vi "Discovery Engine.vi"() -> ()   [LabVIEW 2020]
doc: "This VI broadcasts the IP addresses available on the target on the UDP broadcast address 234.5.6.7, port 58432. It sends this data wrapped in the generic data frame."
uses:
  Type Definitions/Data Frame.ctl
  Type Definitions/Data Frame Header.ctl
  Type Definitions/Payload Class.ctl
  Type Definitions/Device.ctl
  Type Definitions/Discovery Engine State.ctl
  <vilib>/Platform/TimedLoop/XDataNode/timing_clust.ctl
  <vilib>/Platform/TimedLoop/XDataNode/nitl_modes.ctl
  <vilib>/Platform/TimedLoop/XDataNode/wakeup.ctl
  Type Definitions/Network Adapter State.ctl
  Type Definitions/Enum - System State.ctl
  <vilib>/Utility/tcp.llb/UDP Multicast Write-Only Open.vi
  <vilib>/platform/TimedLoop/XDataNode/XDataNode.xnode
  <vilib>/Platform/TimedLoop/XDataNode/XDNodeRunTimeDep.lvlib
panel:
  out "Notifier":refnum<notifier>
  out "Frame":T1 {"CRC" format="%08x"; "Frame Header"."Options" format="%016b"; "Frame Header"."Time" format="%^<%I:%M:%S%3u %p\n%m/%d/%Y %Z>T"; "Frame Header"."Sync" format="%08x"}
  out "Valid IP Addresses":i32
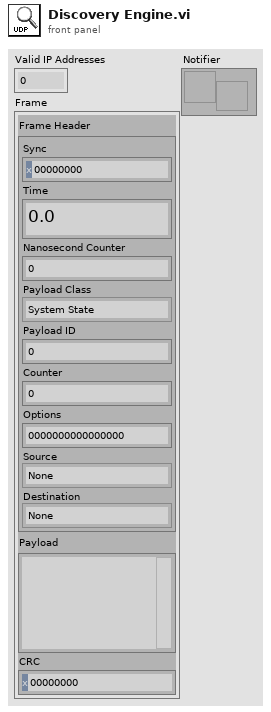
[diagram p1: front panel]
types:
  T1 = typedef "Data Frame.ctl" = cluster{"Frame Header":T2, "Payload":string, "CRC":u32}
  T2 = typedef "Data Frame Header.ctl" = cluster{"Sync":u32, "Time":dbl, "Nanosecond Counter":i64, "Payload Class":T3, "Payload ID":u16, "Counter":i32, "Options":u32, "Source":T4, "Destination":T4}
  T3 = typedef "Payload Class.ctl" = enum16{"System State", "Parameters", "Metadata", "Software Monitor", "Data", "Commands"}
  T4 = typedef "Device.ctl" = enum32{"None", "Exec", "Aux1", "Aux2", "Aux3"}
  T5 = typedef "Discovery Engine State.ctl" = cluster{"Adapter IP Address":string, "Connection ID":refnum<k16>, "Error":errorcluster}
  T6 = typedef "XDNodeRunTimeDep.lvlib/timing_clust.ctl" = cluster{"Expected End [f-1]":u64, "Actual End [f-1]":u64, "Finished Late? [f-1]":bool, "Expected End [i-1]":u64, "Actual End [i-1]":u64, "Finished Late? [i-1]":bool, "Expected Start [i]":u64, "Actual Start [i]":u64, "Expected Start [f]":u64, "Actual Start [f]":u64, "Source Name":string, "Structure Name":string, "Period":i64, "Deadline":i64, "Offset":i64, "Start":i64, "Priority":i32, "Timeout":i32, "Mode":T7, "Wakeup Reason":T8, "Error":errorcluster, "Source Type":string, "Secondary Source Type":string, "Global End Time":u64, "Global Start Time":u64, "Frame Duration":u64, "Iteration Duration":u64, "Assigned CPU":i32, "I/O Scan Engine Mode":u32}
  T7 = typedef "XDNodeRunTimeDep.lvlib/nitl_modes.ctl" = enum32{"No Change", "Process missed periods, maintain original phase", "Discard missed periods, maintain original phase", "Process missed periods, ignore original phase", "Discard missed periods, ignore original phase"}
  T8 = typedef "XDNodeRunTimeDep.lvlib/wakeup.ctl" = enum32{"Normal", "Aborted", "Asynchronous wakeup", "Timing source error", "Timed loop error", "Timeout"}
  T9 = typedef "Enum - System State.ctl" = enum16{"System Time", "Telemetry TCP State", "Writeable Drive State", "Command TCP State", "Network Adapter State", "Discovery Engine State", "Disk State"}
  T10 = typedef "Network Adapter State.ctl" = cluster{"Adapter IP Addresses":string[]}
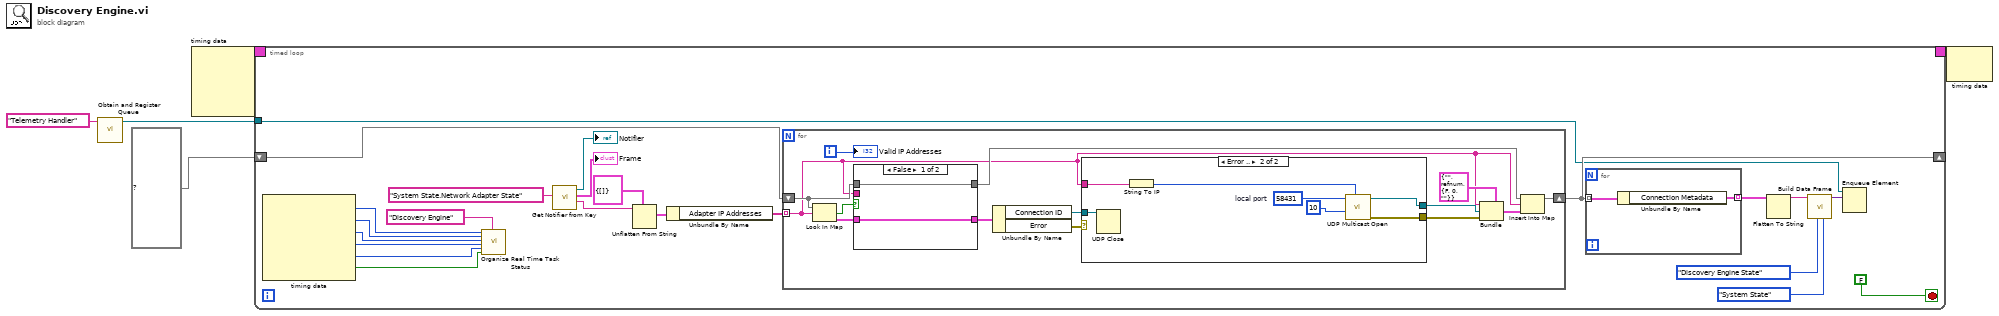
[diagram p0: block diagram]
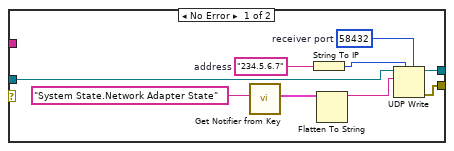
[diagram p2: hidden frame]
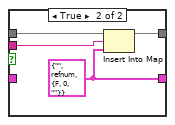
[diagram p3: hidden frame]
diagram:
  n1 = call "Obtain and Register Queue.vi"("name (unnamed)"="Telemetry Handler") -> ("Queue Out"=w3:refnum<queue>)  [unwired: 7 in, 3 out]
  n2 = node-c288() -> (w5:T6)  [unwired: 4 in]
  n3 = timed-loop {
    timing: w5 -> [_]
    timing-out: [_] -> w4
    tunnel: w3 -> [w9]
    shift-right: [w15] -> _
    shift-left: map{string, T5} {} ("map") -> [w16]
    stop <- FALSE stop-if-true
    n4 = node-c288() -> (w26:i32, w25:i32, w24:i64, w23:i64, w22:i64, w21:bool)  [unwired: 1 in]
    n5 = call "Organize Real Time Task Status.vi"("Priority"=w26, "Processor"=w25, "Offset"=w24, "Iteration Duration"=w23, "Period"=w22, "Finished Late? [i-1]"=w21, "Task Name"="Discovery Engine") -> ()  [unwired: 12 in, 1 out]
    n6 = call "Get Notifier from Key.vi"("Notifier Key"="System State.Network Adapter State") -> ("Payload"=w18:string, "Frame"=→"Frame":T1, "Notifier"=→"Notifier":refnum<notifier>)  [unwired: 8 in]
    n7 = Unflatten From String(type=T10 {"Adapter IP Addresses"=[]} ("Network Adapter Metadata"), binary string=w18) -> (value=w20:T10)  [unwired: 3 in, 2 out]
    n8 = Unbundle By Name(w20) -> ("Adapter IP Addresses"=w8:string[])
    n9 = for {
      tunnel: w8 -> [w31] mode=indexing
      shift-right: [w37] -> w15
      shift-left: w16 -> [w43]
      i -> [w34]
      n10 = Look In Map(map=w43, key=w31) -> (key not found?=w44:bool, value=w42:T5)  [unwired: 1 in]
      n11 = case shown="False" w44 {
        tunnel: w43 -> [w62 w66]
        tunnel: w31 -> [_ w65]
        tunnel: [w62 w64] -> w38
        tunnel: w42 -> [w61 _]
        tunnel: [w61 w63] -> w41
        frame False {
        }
        frame True {
          w63 = T5 {"Adapter IP Address"="", "Connection ID"=refnum, "Error"={"status"=FALSE, "code"=0, "source"=""}} ("Connection Metadata")
          n12 = Insert Into Map(map in=w66, key=w65, value=w63) -> (map out=w64:map{string, T5})  [unwired: 2 out]
        }
      }
      n13 = Unbundle By Name(w41) -> ("Connection ID"=w40:refnum<k16>, "Error"=w39:errorcluster)
      n14 = case shown="Error .." w39 {
        tunnel: [w51 w58] -> w33
        tunnel: [w50 w59] -> w32
        tunnel: w40 -> [w49 w60]
        tunnel: w31 -> [_ w54]
        frame No Error {
          w48 = u16 58432  # receiver port
          w46 = "234.5.6.7"  # address
          n15 = call "Get Notifier from Key.vi"("Notifier Key"="System State.Network Adapter State") -> ("Frame"=w52:T1)  [unwired: 8 in, 2 out]
          n16 = String To IP(1:w46) -> (0:w47:u32)
          n17 = Flatten To String(anything=w52) -> (data string=w45:string)  [unwired: 3 in, 2 out]
          n18 = UDP Write(address=w47, port or service name=w48, connection ID=w49, data in=w45) -> (error out=w51:errorcluster, 3:w50:refnum<k16>)  [unwired: 2 in]
        }
        frame Error {
          w57 = u16 58431  # local port
          n19 = UDP Close(connection ID=w60) -> ()  [unwired: 1 in, 2 out]
          n20 = String To IP(1:w54) -> (0:w55:u32)
          n21 = call-poly <vilib>:"UDP Multicast Open.vi"("net address"=w55, "time-to-live (1)"=u16 10, "port"=w57) -> ("error out"=w58:errorcluster, "connection ID"=w59:refnum<k16>)  [unwired: 7 in]
        }
      }
      n22 = Bundle(cluster=T5 {"Adapter IP Address"="", "Connection ID"=refnum, "Error"={"status"=FALSE, "code"=0, "source"=""}} ("Connection Metadata"), "Adapter IP Address"=w31, "Connection ID"=w32, "Error"=w33) -> (w36:T5)
      n23 = Insert Into Map(map in=w38, key=w31, value=w36) -> (map out=w37:map{string, T5})  [unwired: 2 out]
      "Valid IP Addresses" <- w34
    }
    n24 = for {
      tunnel: w15 -> [w30] mode=indexing
      tunnel: [w29] -> w11 mode=indexing
      n25 = Unbundle By Name(w30) -> ("Connection Metadata"=w29:T5)
    }
    n26 = Flatten To String(anything=w11) -> (data string=w14:string)  [unwired: 3 in, 2 out]
    n27 = call "Build Data Frame.vi"("Payload Class (Data)"=Payload_Class."System State", "Payload ID (0)"=Enum_-_System_State."Discovery Engine State" ("System State"), "Payload (Empty String)"=w14) -> ("Frame"=w10:variant)  [unwired: 7 in, 1 out]
    n28 = Enqueue Element(queue=w9, element=w10) -> ()  [unwired: 2 in, 3 out]
  }
  n29 = node-c288(w4) -> ()  [unwired: 1 out]
